vi "TCP Kernel.vi"(6 "HW queue in":refnum<queue>, 8 "error in (no error)":errorcluster, 9 "queue in":refnum<queue>, 10 "Stop Kernel Notifier":refnum<notifier>, 11 "Data indicator":refnum<vi>) -> (0 "error out":errorcluster)   [LabVIEW 2016]
doc: "TCP server. incorporates automatic restart if closed."
uses:
  DataType.ctl
  data_command_enum.ctl
  TCP_enum.ctl
  <vilib>/NI/STM/TCP/TCP Connection Info.ctl
  <vilib>/NI/STM/SubVIs/MetaDataElement.ctl
  <vilib>/NI/STM/TCP/TCP Read Options.ctl
  TCP_Reply_enum.ctl
  <vilib>/NI/STM/TCP/Write Meta Data (TCP Ref).vi
  <vilib>/NI/STM/TCP/Get Connection Reference (TCP).vi
  <vilib>/NI/STM/TCP/Write Meta Data (TCP Clst).vi
  <vilib>/NI/STM/TCP/Write Message (TCP).vi
  <vilib>/NI/STM/TCP/Read Message (TCP).vi
  EK-P4 Global.vi
  <vilib>/NI/STM/NI STM.lvlib
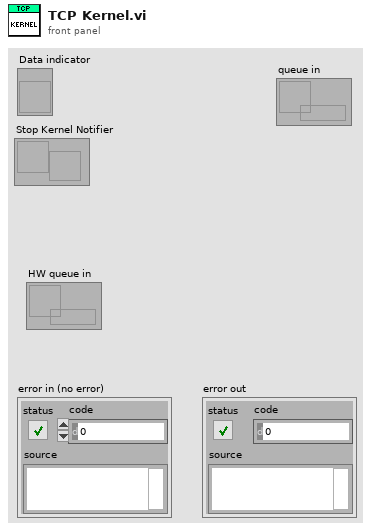
[diagram p1: front panel]
types:
  T1 = typedef "NI STM.lvlib/TCP Connection Info.ctl" = cluster{"connection ID":refnum<k5>, "meta data":T2[]}
  T2 = typedef "NI STM.lvlib/MetaDataElement.ctl" = string
  T3 = cluster{"connection info":T1, "data string":refnum<vi>, "Stop Kernel Notifier":refnum<notifier>, "HW Queue":refnum<queue>}
  T4 = typedef "TCP_enum.ctl" = enum16{"Listen", "Read and Write", "Disconnect", "Exit"}
  T5 = typedef "NI STM.lvlib/TCP Read Options.ctl" = cluster{"ignore timeout error":bool, "timeout ms (1000)":i32}
  T6 = typedef "TCP_Reply_enum.ctl" = enum16{"SendAck", "SendError", "NoAnswer"}
  T7 = typedef "DataType.ctl" = cluster{"command":T8, "data":variant}
  T8 = typedef "data_command_enum.ctl" = enum16{"data", "display", "quit", "save", "filepath", "weak left", "state", "weak right", "strong left", "strong right", "stopRecording", "close", "sid"}
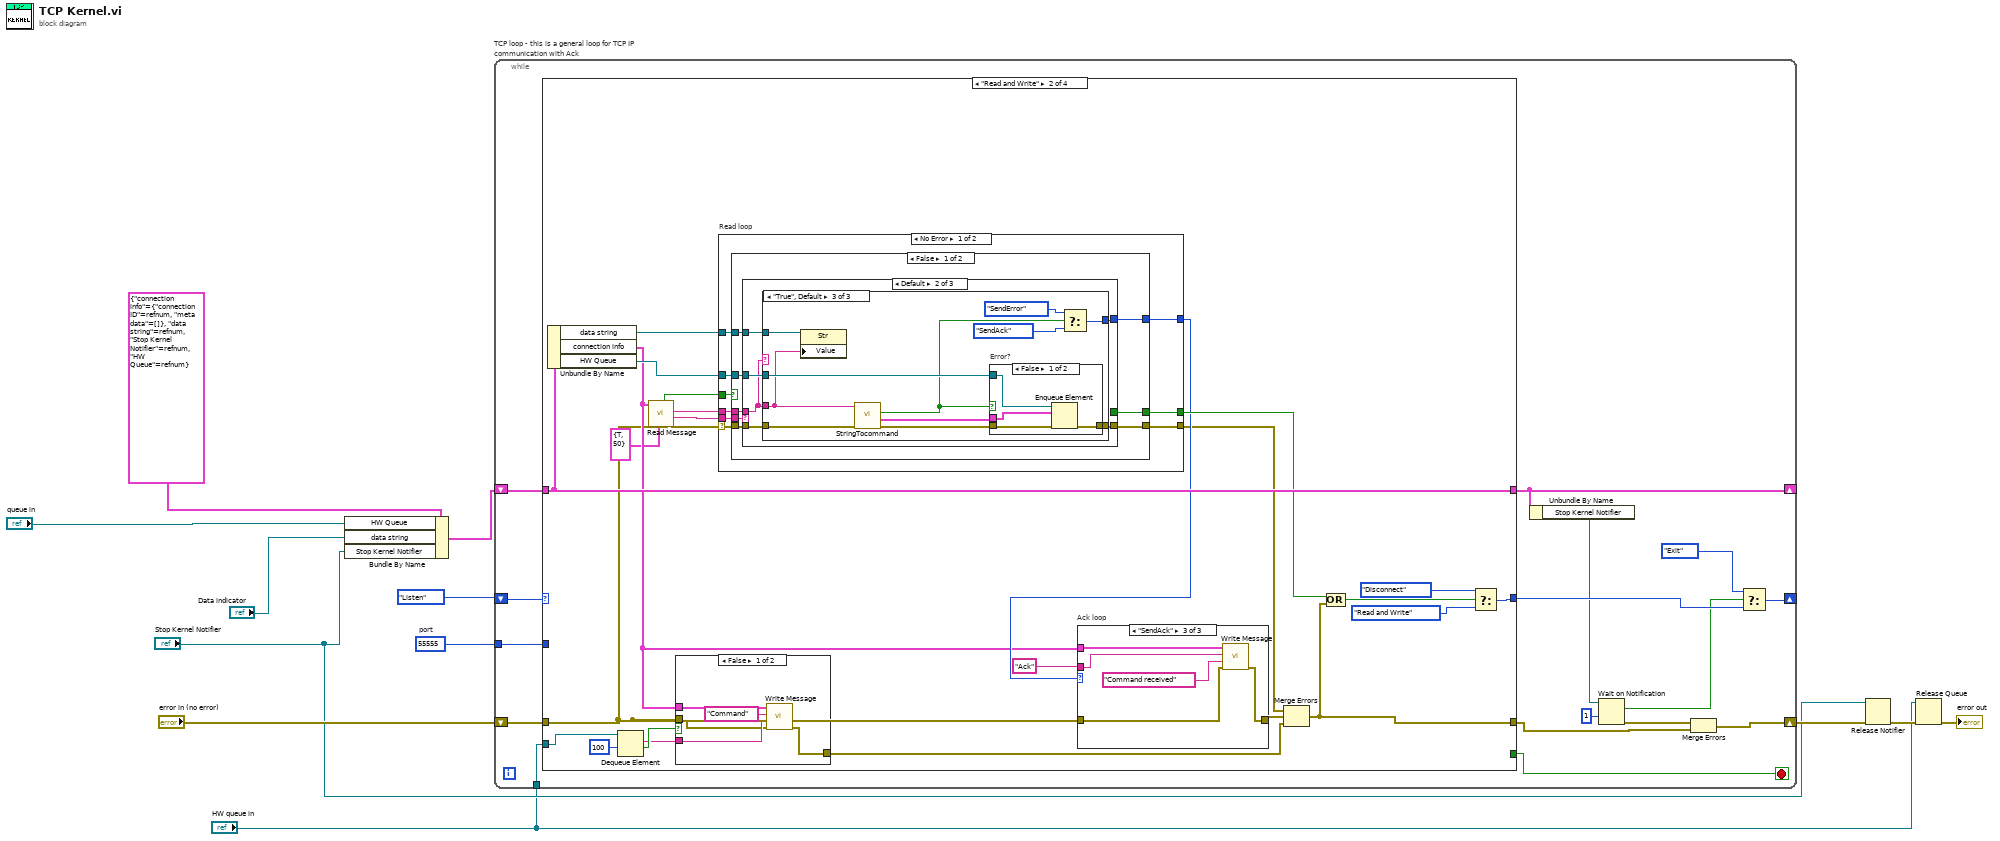
[diagram p0: block diagram]
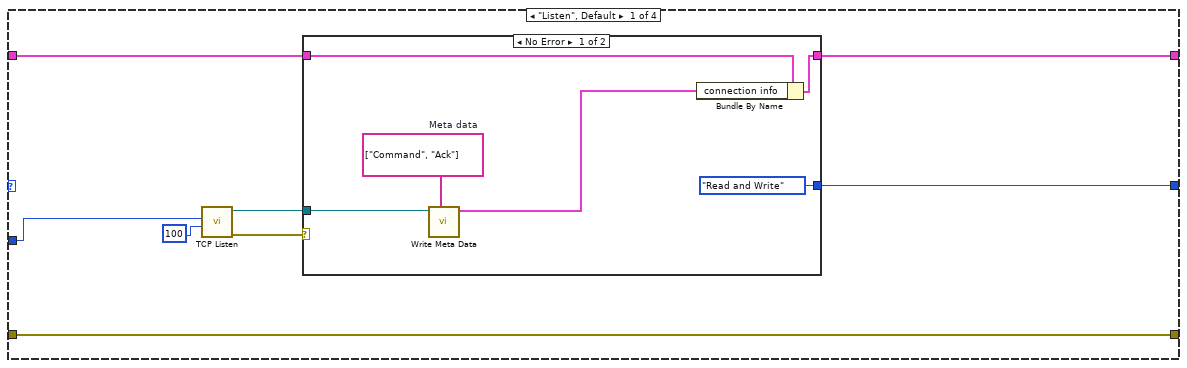
[diagram p2: hidden frame]
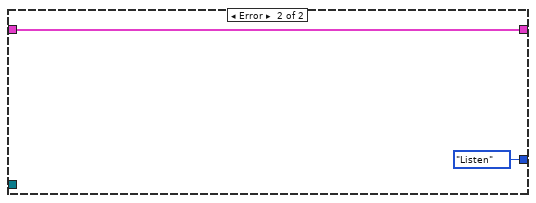
[diagram p3: hidden frame]
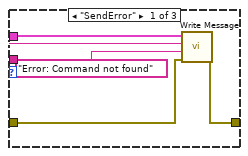
[diagram p5: hidden frame]
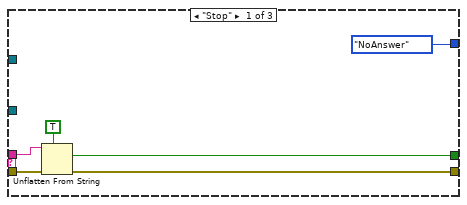
[diagram p7: hidden frame]
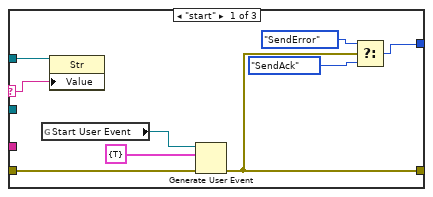
[diagram p8: hidden frame]
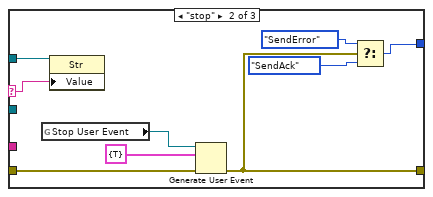
[diagram p9: hidden frame]
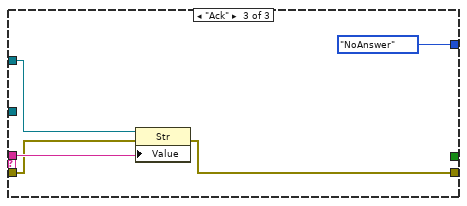
[diagram p11: hidden frame]
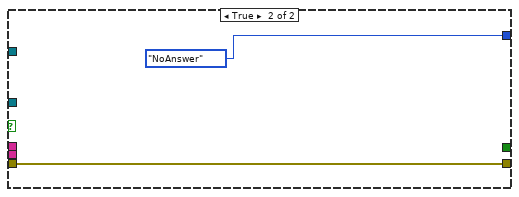
[diagram p12: hidden frame]
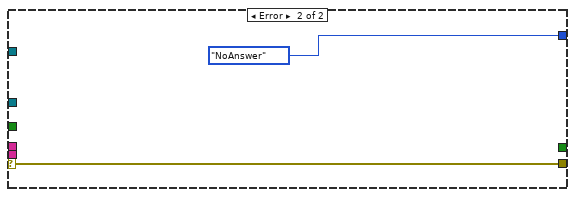
[diagram p13: hidden frame]
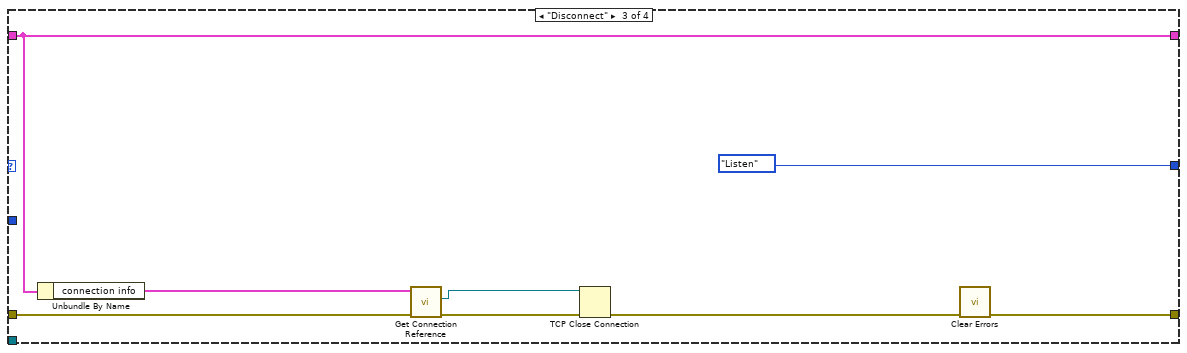
[diagram p14: hidden frame]
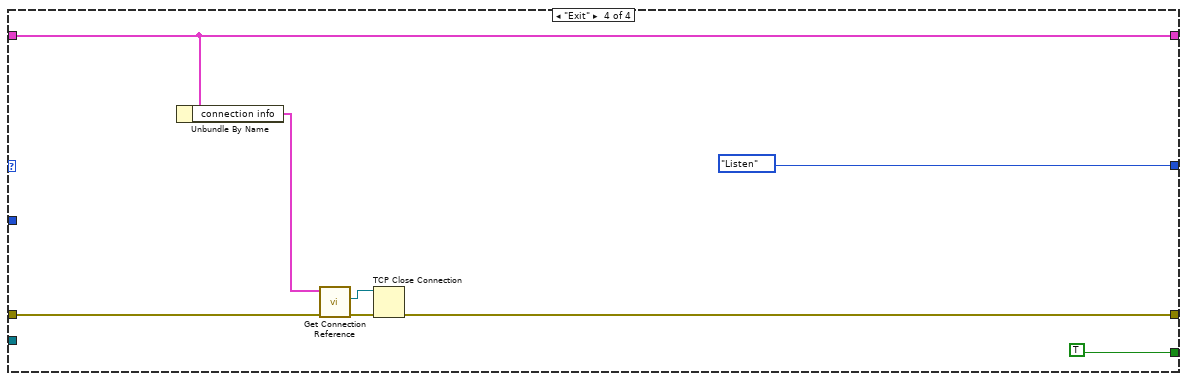
[diagram p15: hidden frame]
diagram:
  w7 = u16 55555  # port
  n1 = Bundle By Name(cluster=T3 {"connection info"={"connection ID"=refnum, "meta data"=[]}, "data string"=refnum, "Stop Kernel Notifier"=refnum, "HW Queue"=refnum}, "HW Queue"="queue in", "data string"="Data indicator", "Stop Kernel Notifier"="Stop Kernel Notifier") -> (w9:T3)
  n2 = while "TCP loop - this is a general loop for TCP IP communication with Ack" {
    tunnel: w7 -> [w27]
    shift-right: [w20] -> _
    shift-left: w9 -> [w26]
    shift-right: [w22] -> _
    shift-left: TCP_enum."Listen" ("TCP States") -> [w28]
    shift-right: [w15] -> w12
    shift-left: "error in (no error)" -> [w25]
    tunnel: "HW queue in" -> [w13]
    stop <- w24 stop-if-true
    n3 = case shown="\"Read and Write\"" w28 {
      tunnel: w27 -> [w35 _ _ _]
      tunnel: w26 -> [w30 w69 w164 w170]
      tunnel: [w33 w69 w164 w170] -> w20
      tunnel: [w32 w60 TCP_enum."Listen" ("TCP States") TCP_enum."Listen" ("TCP States")] -> w23
      tunnel: w25 -> [w31 w47 w161 w171]
      tunnel: [w31 w54 w159 w167] -> w14
      tunnel: [_ _ _ TRUE] -> w24
      tunnel: w13 -> [_ w52 _ _]
      frame "Listen", Default {
        n4 = call <vilib>:"TCP Listen.vi"("timeout ms (wait forever: -1)"=100, "port"=w35) -> ("error out"=w29:errorcluster, "connection ID"=w34:refnum<k5>)  [unwired: 2 in, 6 out]
        n5 = case shown="No Error" w29 {
          tunnel: w34 -> [w41 _]
          tunnel: w30 -> [w40 w44]
          tunnel: [w39 w44] -> w33
          tunnel: [TCP_enum."Read and Write" ("TCP States") TCP_enum."Listen" ("TCP States")] -> w32
          frame No Error {
            w42 = T2[] ["Command", "Ack"]  # Meta data
            n6 = call-poly <vilib>:"Write Meta Data.vi"("meta data"=w42, "connection ID"=w41) -> ("connection info out"=w38:T1)  [unwired: 3 in, 6 out]
            n7 = Bundle By Name(cluster=w40, "connection info"=w38) -> (w39:T3)
          }
          frame Error {
          }
        }
      }
      frame "Read and Write" {
        n8 = Unbundle By Name(w69) -> ("data string"=w53:refnum<vi>, "connection info"=w49:T1, "HW Queue"=w59:refnum<queue>)
        n9 = Dequeue Element(queue=w52, timeout in ms (-1)=100) -> (element=w48:string, timed out?=w50:bool)  [unwired: 1 in, 2 out]
        n10 = call-poly <vilib>:"Read Message.vi"("options"=T5 {"ignore timeout error"=TRUE, "timeout ms (1000)"=50}, "error in"=w47, "connection info in"=w49) -> ("error out"=w65:errorcluster, "name"=w68:T2, "data string"=w67:string, "timed out?"=w66:bool)  [unwired: 2 in, 3 out]
        n11 = case shown="False" w50 {
          tunnel: w49 -> [w74 _]
          tunnel: w48 -> [w72 _]
          tunnel: w47 -> [w71 w75]
          tunnel: [w70 w75] -> w46
          frame False {
            n12 = call-poly <vilib>:"Write Message.vi"("error in"=w71, "data"=w72, "name"="Command", "connection info in"=w74) -> ("error out"=w70:errorcluster)  [unwired: 6 in, 1 out]
          }
          frame True {
          }
        }
        n13 = case "Read loop" shown="No Error" w65 {
          selector: w65 -> [w92 w158]
          tunnel: w68 -> [w95 _]
          tunnel: w67 -> [w94 _]
          tunnel: w66 -> [w93 _]
          tunnel: [w91 w158] -> w56
          tunnel: [w90 _] -> w64
          tunnel: w59 -> [w89 _]
          tunnel: [w88 TCP_Reply_enum."NoAnswer" ("Reply")] -> w57
          tunnel: w53 -> [w87 _]
          frame No Error {
            n14 = case shown="False" w93 {
              tunnel: w95 -> [w100 _]
              tunnel: w94 -> [w103 _]
              tunnel: w92 -> [w102 w156]
              tunnel: [w101 w156] -> w91
              tunnel: [w99 _] -> w90
              tunnel: w89 -> [w98 _]
              tunnel: [w97 TCP_Reply_enum."NoAnswer" ("Reply")] -> w88
              tunnel: w87 -> [w96 _]
              frame False {
                n15 = case shown="Default" w100 {
                  tunnel: w103 -> [w108 w110 w153]
                  tunnel: w102 -> [w107 w113 w151]
                  tunnel: [w104 w115 w150] -> w101
                  tunnel: [w106 _ _] -> w99
                  tunnel: w98 -> [_ w114 _]
                  tunnel: [TCP_Reply_enum."NoAnswer" ("Reply") w112 TCP_Reply_enum."NoAnswer" ("Reply")] -> w97
                  tunnel: w96 -> [_ w111 w152]
                  frame "Stop" {
                    n16 = Unflatten From String(type=TRUE, binary string=w108, error in (no error)=w107) -> (value=w106:bool, error out=w104:errorcluster)  [unwired: 1 in, 2 out]
                  }
                  frame Default {
                    n17 = case shown="\"True\", Default" w110 {
                      selector: w110 -> [w121 w130 _]
                      tunnel: [w117 w126 w144] -> w115
                      tunnel: w114 -> [_ _ w143]
                      tunnel: w113 -> [w118 w127 w142]
                      tunnel: [w116 w125 w136] -> w112
                      tunnel: w111 -> [w122 w131 w135]
                      tunnel: w110 -> [_ _ w134]
                      frame "start" {
                        n18 = global read "EK-P4 Global.vi" "Start User Event"() -> (w120:refnum<user-event>)
                        n19 = property class="Str"(reference=w122, "Value"=w121) -> ()  [unwired: 1 in, 2 out]
                        n20 = Generate User Event(user event=w120, event data cluster=cluster{bool} {TRUE} ("event data"), error in=w118) -> (error out=w117:errorcluster)  [unwired: 1 in, 1 out]
                        n21 = Select(t=TCP_Reply_enum."SendError" ("Reply"), s=w117, f=TCP_Reply_enum."SendAck" ("Reply")) -> (s? t:f=w116:T6)
                      }
                      frame "stop" {
                        n22 = global read "EK-P4 Global.vi" "Stop User Event"() -> (w129:refnum<user-event>)
                        n23 = property class="Str"(reference=w131, "Value"=w130) -> ()  [unwired: 1 in, 2 out]
                        n24 = Generate User Event(user event=w129, event data cluster=cluster{bool} {TRUE} ("event data"), error in=w127) -> (error out=w126:errorcluster)  [unwired: 1 in, 1 out]
                        n25 = Select(t=TCP_Reply_enum."SendError" ("Reply"), s=w126, f=TCP_Reply_enum."SendAck" ("Reply")) -> (s? t:f=w125:T6)
                      }
                      frame "True", Default {
                        n26 = property class="Str"(reference=w135, "Value"=w134) -> ()  [unwired: 1 in, 2 out]
                        n27 = call "StringTocommand.vi"("error in"=w142, "data string"=w134) -> ("error out"=w141:errorcluster, "output cluster"=w140:T7, "Error?"=w139:bool)  [unwired: 5 in, 2 out]
                        n28 = case "Error?" shown="False" w139 {
                          tunnel: [w148 w149] -> w144
                          tunnel: w143 -> [w147 _]
                          tunnel: w141 -> [w146 w149]
                          tunnel: w140 -> [w145 _]
                          frame False {
                            n29 = Enqueue Element(queue=w147, element=w145, error in (no error)=w146) -> (error out=w148:errorcluster)  [unwired: 1 in, 2 out]
                          }
                          frame True {
                          }
                        }
                        n30 = Select(t=TCP_Reply_enum."SendError" ("Reply"), s=w139, f=TCP_Reply_enum."SendAck" ("Reply")) -> (s? t:f=w136:T6)
                      }
                    }
                  }
                  frame "Ack" {
                    n31 = property class="Str"(reference=w152, error in=w151, "Value"=w153) -> (error out=w150:errorcluster)  [unwired: 1 out]
                  }
                }
              }
              frame True {
              }
            }
          }
          frame Error {
          }
        }
        n32 = case "Ack loop" shown="\"SendAck\"" w57 {
          tunnel: w47 -> [w77 w81 w83]
          tunnel: w49 -> [w80 _ w86]
          tunnel: "Ack" ("name") -> [w79 _ w85]
          tunnel: [w76 w81 w82] -> w55
          frame "SendError" {
            n33 = call-poly <vilib>:"Write Message.vi"("error in"=w77, "data"="Error: Command not found", "name"=w79, "connection info in"=w80) -> ("error out"=w76:errorcluster)  [unwired: 6 in, 1 out]
          }
          frame "NoAnswer", Default {
          }
          frame "SendAck" {
            n34 = call-poly <vilib>:"Write Message.vi"("error in"=w83, "data"="Command received", "name"=w85, "connection info in"=w86) -> ("error out"=w82:errorcluster)  [unwired: 6 in, 1 out]
          }
        }
        n35 = Merge Errors(w56, w55, w46) -> (w54:errorcluster)
        n36 = Compound Arithmetic op=OR(w64, w54) -> (w63:bool)
        n37 = Select(t=TCP_enum."Disconnect" ("TCP States"), s=w63, f=TCP_enum."Read and Write" ("TCP States")) -> (s? t:f=w60:T4)
      }
      frame "Disconnect" {
        n38 = Unbundle By Name(w164) -> ("connection info"=w163:T1)
        n39 = call-poly <vilib>:"Get Connection Reference.vi"("error in"=w161, "connection info in"=w163) -> ("error out"=w165:errorcluster, "connection ID out"=w166:refnum<k5>)  [unwired: 8 out]
        n40 = TCP Close Connection(connection ID=w166, error in (no error)=w165) -> (error out=w160:errorcluster)  [unwired: 2 out]
        n41 = call <vilib>:"Clear Errors.vi"("error in (no error)"=w160) -> ("error out"=w159:errorcluster)  [unwired: 5 in, 1 out]
      }
      frame "Exit" {
        n42 = Unbundle By Name(w170) -> ("connection info"=w169:T1)
        n43 = call-poly <vilib>:"Get Connection Reference.vi"("error in"=w171, "connection info in"=w169) -> ("error out"=w172:errorcluster, "connection ID out"=w173:refnum<k5>)  [unwired: 8 out]
        n44 = TCP Close Connection(connection ID=w173, error in (no error)=w172) -> (error out=w167:errorcluster)  [unwired: 2 out]
      }
    }
    n45 = Unbundle By Name(w20) -> ("Stop Kernel Notifier"=w18:refnum<notifier>)
    n46 = Wait on Notification(notifier=w18, timeout in ms (-1)=1) -> (notification=w16:bool, error out=w19:errorcluster)  [unwired: 2 in, 2 out]
    n47 = Merge Errors(w19, w14) -> (w15:errorcluster)
    n48 = Select(t=TCP_enum."Exit" ("TCP States"), s=w16, f=w23) -> (s? t:f=w22:T4)
  }
  n49 = Release Notifier(notifier="Stop Kernel Notifier", error in (no error)=w12) -> (error out=w5:errorcluster)  [unwired: 1 in, 2 out]
  n50 = Release Queue(queue="HW queue in", error in (no error)=w5) -> (error out=→"error out":errorcluster)  [unwired: 1 in, 2 out]
